vi "Excel_Insert_Textbox.vi"(0 "Excel.Shapes":refnum<k7>, 1 "font":T2 {"font size" format="%0.2f"; "strike through" items=["Strk Unchanged", "Strk Yes", "Strk No"]; "underline" items=["Und Unchanged", "Und Yes", "Und No"]; "italic" items=["Ital Unchanged", "Ital Yes", "Ital No"]; "bold" items=["Bold Unchanged", "Bold Yes", "Bold No"]}, 2 "frame visible?":bool, 5 "Excel._Worksheet":refnum<k7>, 7 "orientation":i32(ring)=1 items=["msoTextOrientationMixed"=-2, "msoTextOrientationHorizontal"=1, "msoTextOrientationUpward"=2, "msoTextOrientationDownward"=3, "msoTextOrientationVerticalFarEast"=4, "msoTextOrientationVertical"=5, "msoTextOrientationHorizontalRotatedFarEast"=6], 9 "text":string, 11 "error in (no error)":errorcluster, 12 "position/size":T1 {"Height" format="%0.2f"; "Width" format="%0.2f"}, 13 "measurement system":u16(ring) caption="measurement system (US)", 14 "name":string) -> (15 "error out":errorcluster)   [LabVIEW 2010, in "NI_ReportGenerationToolkit.lvlib"]
uses:
  <vilib>/addons/_office/NI_ReportGenerationToolkit.lvlib
  <vilib>/addons/_office/_exclsub.llb/font.ctl
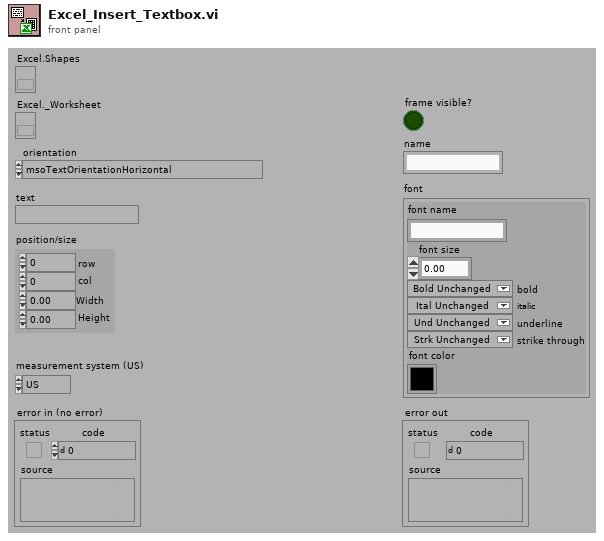
[diagram p1: front panel]
types:
  T1 = cluster{"row":i32, "col":i32, "Width":dbl, "Height":dbl}
  T2 = typedef "NI_ReportGenerationToolkit.lvlib/font.ctl" = cluster{"font name":string, "font size":dbl, "bold":u16, "italic":u16, "underline":u16, "strike through":u16, "font color":u32}
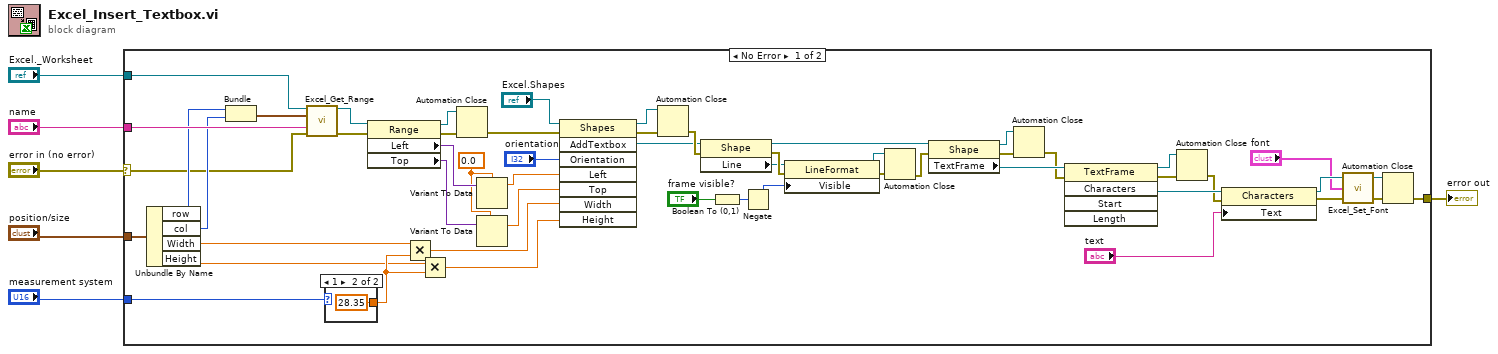
[diagram p0: block diagram]
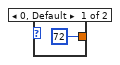
[diagram p2: hidden frame]
diagram:
  n1 = case shown="No Error" "error in (no error)" {
    selector: "error in (no error)" -> [w8 w62]
    tunnel: "position/size" -> [w50 _]
    tunnel: "measurement system" -> [w29 _]
    tunnel: [w24 w62] -> w4
    tunnel: "Excel._Worksheet" -> [w13 _]
    tunnel: "name" -> [w12 _]
    frame No Error {
      w47 = sgl 0.0 ("Left")
      n2 = Unbundle By Name(w50) -> ("row"=w11:i32, "col"=w10:i32, "Width"=w51:dbl, "Height"=w52:dbl)
      n3 = Bundle("row"=w11, "col"=w10) -> (w9:cluster{"row":i32, "col":i32})  [unwired: 1 out]
      n4 = call <vilib>:"Excel_Get_Range.vi"("Excel._Worksheet"=w13, "start"=w9, "name"=w12, "error in (no error)"=w8) -> ("Range"=w7:refnum<k7>, "error out"=w14:errorcluster)  [unwired: 1 in, 9 out]
      n5 = case shown="1" w29 {
        tunnel: [72 28.35] -> w53
        frame 0, Default {
        }
        frame 1 {
        }
      }
      n6 = property class="Range"(reference=w7, error in=w14) -> (reference out=w46:refnum<k7>, error out=w45:errorcluster, "Left"=w48:variant, "Top"=w49:variant)
      n7 = Multiply(x=w51, y=w53) -> (x*y=w56:dbl)
      n8 = Multiply(x=w52, y=w53) -> (x*y=w57:dbl)
      n9 = Automation Close(3:w45, 5:w46) -> (0:w59:errorcluster)
      n10 = Variant To Data(Variant=w48, type=w47) -> (data=w54:sgl)  [unwired: 1 in, 1 out]
      n11 = Variant To Data(Variant=w49, type=w47) -> (data=w55:sgl)  [unwired: 1 in, 1 out]
      n12 = invoke class="Shapes" method="AddTextbox"(reference="Excel.Shapes", error in=w59, "Orientation"="orientation", "Left"=w54, "Top"=w55, "Width"=w56, "Height"=w57) -> (reference out=w23:refnum<k7>, error out=w22:errorcluster, "AddTextbox"=w33:refnum<k7>)  [unwired: 1 in, 5 out]
      n13 = Automation Close(3:w22, 5:w23) -> (0:w35:errorcluster)
      n14 = property class="Shape"(reference=w33, error in=w35) -> (reference out=w34:refnum<k7>, error out=w36:errorcluster, "Line"=w32:refnum<k7>)
      n15 = Boolean To (0,1)(Boolean="frame visible?") -> (0, 1=w42:i16)
      n16 = Negate(x=w42) -> (-x=w43:i16)
      n17 = property class="LineFormat"(reference=w32, error in=w36, "Visible"=w43) -> (reference out=w40:refnum<k7>, error out=w39:errorcluster)
      n18 = Automation Close(3:w39, 5:w40) -> (0:w41:errorcluster)
      n19 = property class="Shape"(reference=w34, error in=w41) -> (reference out=w38:refnum<k7>, error out=w37:errorcluster, "TextFrame"=w31:refnum<k7>)
      n20 = Automation Close(3:w37, 5:w38) -> (0:w18:errorcluster)
      n21 = invoke class="TextFrame" method="Characters"(reference=w31, error in=w18) -> (reference out=w15:refnum<k7>, error out=w17:errorcluster, "Characters"=w21:refnum<k7>)  [unwired: 3 in, 2 out]
      n22 = Automation Close(3:w17, 5:w15) -> (0:w16:errorcluster)
      n23 = property class="Characters"(reference=w21, error in=w16, "Text"="text") -> (reference out=w30:refnum<k7>, error out=w25:errorcluster)
      n24 = call <vilib>:"Excel_Set_Font.vi"("Excel.Characters"=w30, "font"="font", "error in (no error)"=w25) -> ("Excel.Characters out"=w27:refnum<k7>, "error out"=w26:errorcluster)  [unwired: 5 out]
      n25 = Automation Close(3:w26, 5:w27) -> (0:w24:errorcluster)
    }
    frame Error {
    }
  }
  "error out" <- w4
